vi "ArmControlTeleOp.vi"(9 "Robot":T1, 10 "Axes":dbl[](array[numeric]), 11 "Buttons":bool[](array[boolean])) -> ()   [LabVIEW 2015]
uses:
  Robot Type Def.ctl
  Framework/JoystickMappingNamesTypeDef.ctl
  LowShooter/Implementation/Shooter Global.vi
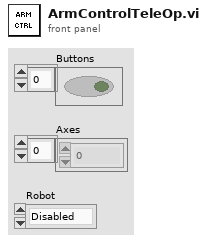
[diagram p1: front panel]
types:
  T1 = typedef "Robot Type Def.ctl" = enum32{"Disabled", "Ghost", "Casper", "Lofty", "Board", "RaceRobot", "Casper 2.0", "Excalibot 2.0"}
  T2 = typedef "JoystickMappingNamesTypeDef.ctl" = enum16{"Shoot Button", "Retrieve Button", "Arm Control", "High Gear", "Low Gear", "Enable PTO", "Disable PTO", "PortC Control", "PortC Up", "PortC Down", "Lift Control", "Drive VBus"}
  T3 = typedef "Arm Settings Type Def.ctl" = cluster{"Min Arm Pos":dbl, "Max Arm Pos":dbl, "Drive Pos":dbl, "Arm Increments":dbl, "Obstacle Pos":dbl}
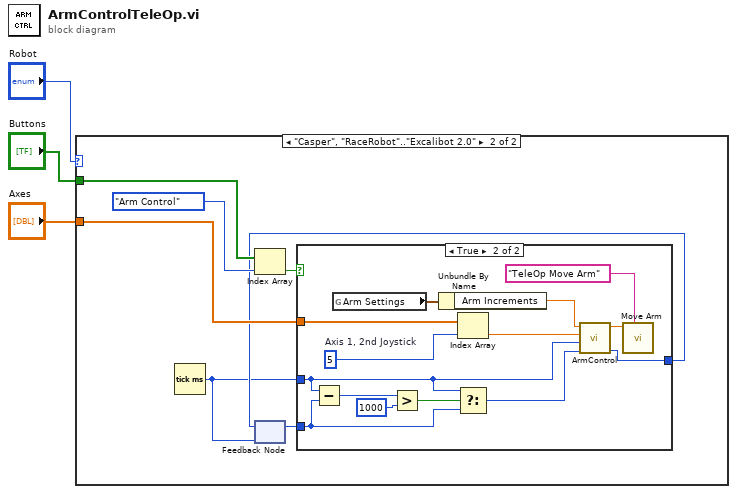
[diagram p0: block diagram]
diagram:
  n1 = case shown="\"Casper\", \"RaceRobot\"..\"Excalibot 2.0\"" "Robot" {
    tunnel: "Buttons" -> [_ w10]
    tunnel: "Axes" -> [_ w8]
    frame "Disabled", Default {
    }
    frame "Casper", "RaceRobot".."Excalibot 2.0" {
      # "Go Up if 4"
      n2 = Tick Count (ms)() -> (millisecond timer value=w4:u32)
      n3 = Index Array(array=w10, index=JoystickMappingNamesTypeDef."Arm Control" ("Joystick Button Names")) -> (element=w7:bool)
      n4 = feedback #1(w4) -> (w5:u32)
      n5 = case shown="True" w7 {
        tunnel: w8 -> [_ w24]
        tunnel: [w11 w20] -> w6
        tunnel: w5 -> [_ w16]
        tunnel: w4 -> [w11 w12]
        frame False {
        }
        frame True {
          w25 = 5  # Axis 1, 2nd Joystick
          n6 = Subtract(x=w12, y=w16) -> (x-y=w19:u32)
          n7 = global read "Shooter Global.vi" "Arm Settings"() -> (w14:T3)
          n8 = Greater?(x=w19, y=u32 1000) -> (0:w17:bool)
          n9 = Unbundle By Name(w14) -> ("Arm Increments"=w13:dbl)
          n10 = Index Array(array=w24, index=w25) -> (element=w23:dbl)
          n11 = Select(t=w12, s=w17, f=w16) -> (s? t:f=w15:u32)
          n12 = call "ArmControl.vi"("Last Increment time"=w15, "Current time"=w12, "Joystick"=w23, "Increment"=w13) -> ("Last Time"=w20:u32, "Increment Amount"=w22:dbl)  [unwired: 6 in]
          n13 = call "Move Arm.vi"("Description"="TeleOp Move Arm", "Angle Increment"=w22) -> ()  [unwired: 8 in, 2 out]
        }
      }
      n14 = feedback-in #1(w6) -> ()
    }
  }
